vi "binarization.vi"() -> ()   [LabVIEW 2024]
uses:
  <vilib>/vision/NI_Vision_Development_Module.lvlib
panel:
  out "SEGMENTED":T1(plugin-control)
  out "error out 4":errorcluster
  out "RED-PLANE":T1(plugin-control)
  out "EQHP":T1(plugin-control)
  out "EQ-LAP":T1(plugin-control)
  out "LAPLAZ":T2(graph)
  out "HIGHP":T2(graph)
  out "LAPL":T1(plugin-control)
  out "FILL LAPLAZ":T1(plugin-control)
  in  "Range 3":cluster{"Lower value":sgl, "Upper value":sgl}={"Lower value"=128.0, "Upper value"=255.0} {"Upper value" format="%.2f"; "Lower value" format="%.2f"}
  out "HIGHPASS":T1(plugin-control)
  out "FILL HIGHPASS":T1(plugin-control)
  in  "Range 2":cluster{"Lower value":sgl, "Upper value":sgl}={"Lower value"=128.0, "Upper value"=255.0} {"Upper value" format="%.2f"; "Lower value" format="%.2f"}
  out "GAUSS":T1(plugin-control)
  out "High-pass":T1(plugin-control)
  out "Laplacian":T1(plugin-control)
  out "Gray":T1(plugin-control)
  out "Equalized":T1(plugin-control)
  out "Waveform Graph 2":T2(graph)
  out "Waveform Graph":T2(graph)
  out "Threshold":T1(plugin-control)
  out "EQUALI":T1(plugin-control)
  out "FILL EQUA":T1(plugin-control)
  in  "Range":cluster{"Lower value":sgl, "Upper value":sgl}={"Lower value"=128.0, "Upper value"=255.0} {"Upper value" format="%.2f"; "Lower value" format="%.2f"}
  out "error out 2":errorcluster
  in  "stop":bool
  out "Select ROI ->  IZQUIERDO":T1(plugin-control)
  out "Ojo Izquierdo":T1(plugin-control)
  out "error out":errorcluster
  out "error out 3":errorcluster
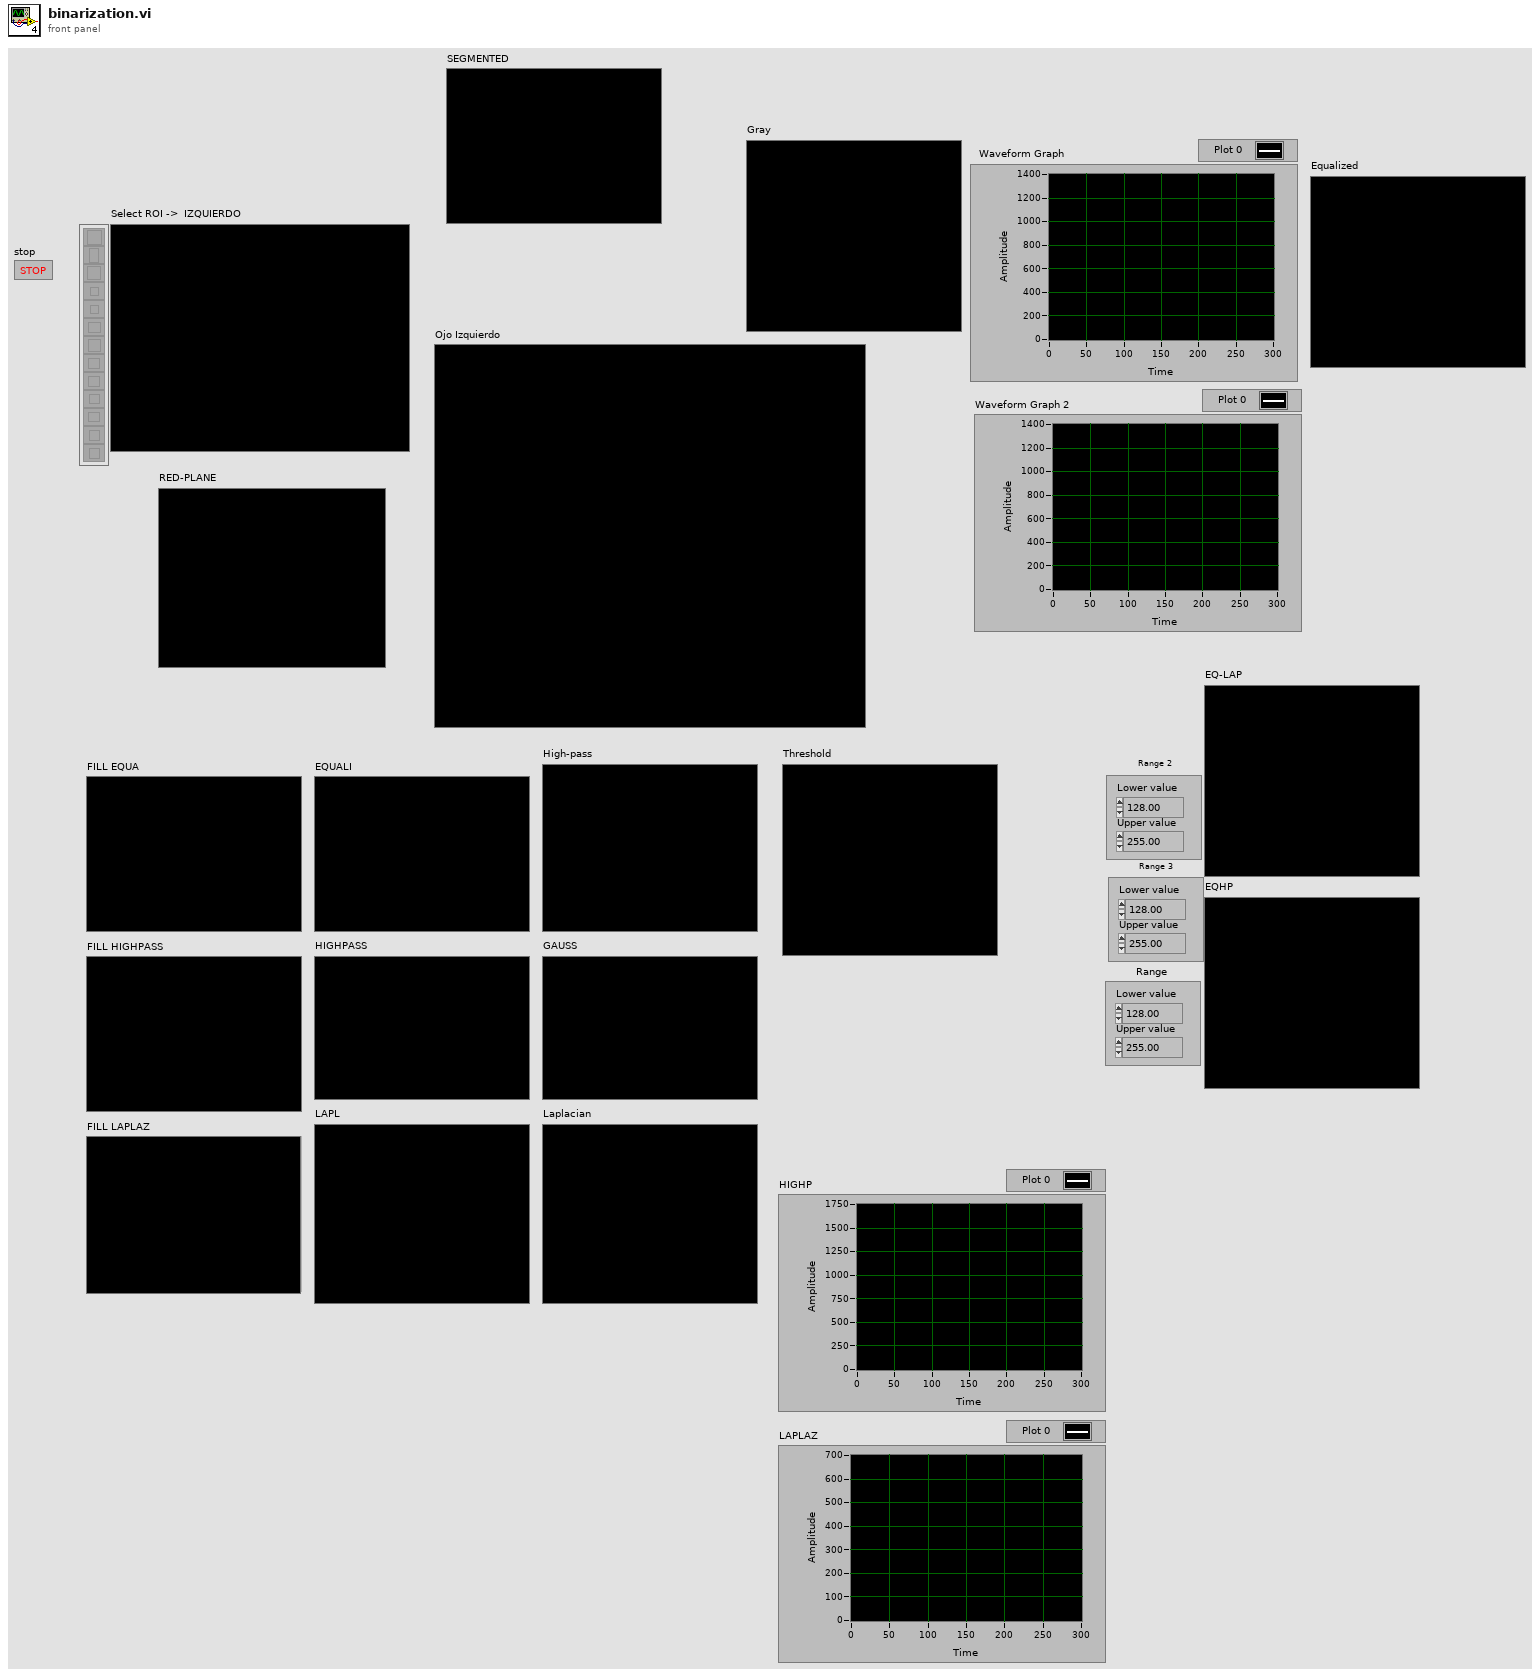
[diagram p1: front panel]
types:
  T1 = typedef "IMAQ Image.ctl" = refnum<image>
  T2 = cluster{"Starting Value":sgl, "Incremental Value":sgl, "Histogram":u32[]}
  T3 = typedef "Image Type" = u32
  T4 = cluster{"Global Rectangle":i32[], "Contours":cluster{"Contour Type":u32, "ROI Type":u32, "Points":i32[]}[]}
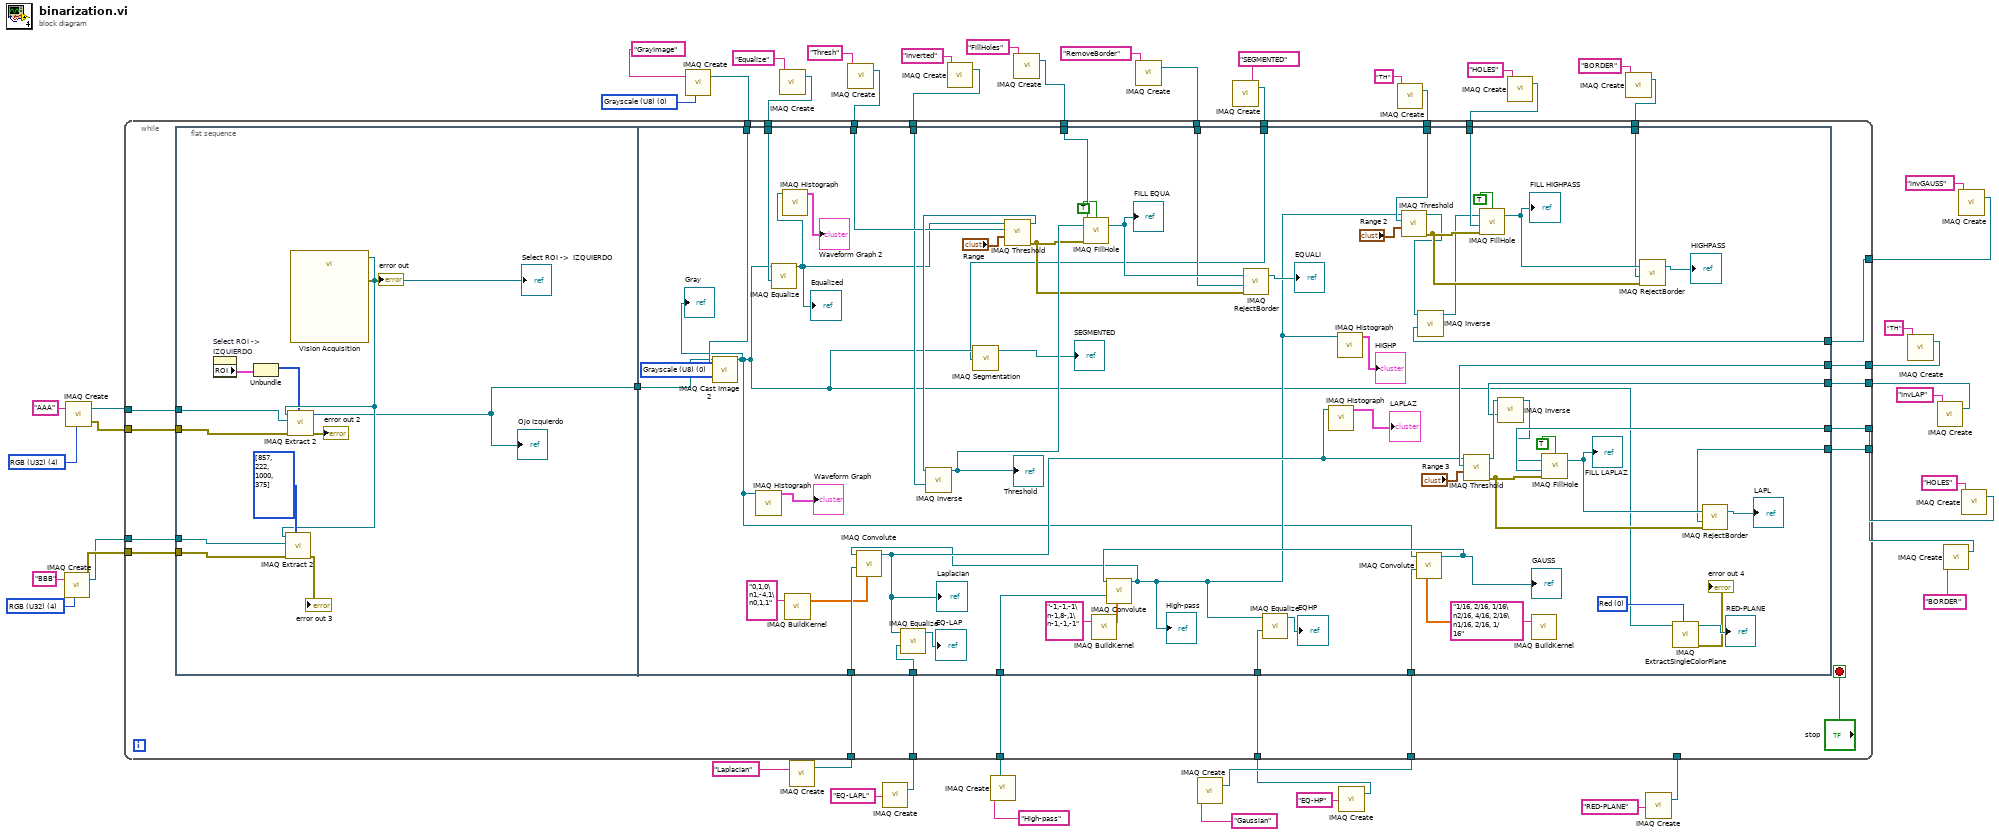
[diagram p0: block diagram]
diagram:
  w42 = T3 0 items=["Grayscale (U8)", "Grayscale (I16)", "Grayscale (SGL)", "Complex (CSG)", "RGB (U32)", "HSL (U32)", "RGB (U64)", "Grayscale (U16)"] ("Image Type")
  w46 = T3 4 items=["Grayscale (U8)", "Grayscale (I16)", "Grayscale (SGL)", "Complex (CSG)", "RGB (U32)", "HSL (U32)", "RGB (U64)", "Grayscale (U16)"] ("Image Type")
  w44 = T3 4 items=["Grayscale (U8)", "Grayscale (I16)", "Grayscale (SGL)", "Complex (CSG)", "RGB (U32)", "HSL (U32)", "RGB (U64)", "Grayscale (U16)"] ("Image Type")
  n1 = call "IMAQ Create"("Image Name"="BBB", "Image Type"=w46) -> ("New Image"=w50:T1, "error out"=w51:errorcluster)  [unwired: 3 in]
  n2 = call "IMAQ Create"("Image Name"="AAA", "Image Type"=w44) -> ("New Image"=w48:T1, "error out"=w49:errorcluster)  [unwired: 3 in]
  n3 = call "IMAQ Create"("Image Name"="GrayImage", "Image Type"=w42) -> ("New Image"=w41:T1)  [unwired: 3 in, 1 out]
  n4 = call "IMAQ Create"("Image Name"="Equalize") -> ("New Image"=w31:T1)  [unwired: 4 in, 1 out]
  n5 = call "IMAQ Create"("Image Name"="Laplacian") -> ("New Image"=w29:T1)  [unwired: 4 in, 1 out]
  n6 = call "IMAQ Create"("Image Name"="Thresh") -> ("New Image"=w36:T1)  [unwired: 4 in, 1 out]
  n7 = call "IMAQ Create"("Image Name"="EQ-LAPL") -> ("New Image"=w7:T1)  [unwired: 4 in, 1 out]
  n8 = call "IMAQ Create"("Image Name"="Inverted") -> ("New Image"=w35:T1)  [unwired: 4 in, 1 out]
  n9 = call "IMAQ Create"("Image Name"="High-pass") -> ("New Image"=w27:T1)  [unwired: 4 in, 1 out]
  n10 = call "IMAQ Create"("Image Name"="FillHoles") -> ("New Image"=w34:T1)  [unwired: 4 in, 1 out]
  n11 = call "IMAQ Create"("Image Name"="RemoveBorder") -> ("New Image"=w33:T1)  [unwired: 4 in, 1 out]
  n12 = call "IMAQ Create"("Image Name"="Gaussian") -> ("New Image"=w25:T1)  [unwired: 4 in, 1 out]
  n13 = call "IMAQ Create"("Image Name"="SEGMENTED") -> ("New Image"=w1:T1)  [unwired: 4 in, 1 out]
  n14 = call "IMAQ Create"("Image Name"="EQ-HP") -> ("New Image"=w5:T1)  [unwired: 4 in, 1 out]
  n15 = call "IMAQ Create"("Image Name"="TH") -> ("New Image"=w21:T1)  [unwired: 4 in, 1 out]
  n16 = call "IMAQ Create"("Image Name"="HOLES") -> ("New Image"=w20:T1)  [unwired: 4 in, 1 out]
  n17 = call "IMAQ Create"("Image Name"="BORDER") -> ("New Image"=w19:T1)  [unwired: 4 in, 1 out]
  n18 = call "IMAQ Create"("Image Name"="RED-PLANE") -> ("New Image"=w3:T1)  [unwired: 4 in, 1 out]
  n19 = call "IMAQ Create"("Image Name"="TH") -> ("New Image"=w15:T1)  [unwired: 4 in, 1 out]
  n20 = call "IMAQ Create"("Image Name"="invLAP") -> ("New Image"=w11:T1)  [unwired: 4 in, 1 out]
  n21 = call "IMAQ Create"("Image Name"="BORDER") -> ("New Image"=w13:T1)  [unwired: 4 in, 1 out]
  n22 = call "IMAQ Create"("Image Name"="invGAUSS") -> ("New Image"=w9:T1)  [unwired: 4 in, 1 out]
  n23 = call "IMAQ Create"("Image Name"="HOLES") -> ("New Image"=w14:T1)  [unwired: 4 in, 1 out]
  n24 = while {
    tunnel: w48 -> [w75]
    tunnel: w49 -> [w76]
    tunnel: w50 -> [w74]
    tunnel: w51 -> [w73]
    tunnel: w41 -> [w72]
    tunnel: w36 -> [w70]
    tunnel: w35 -> [w69]
    tunnel: w34 -> [w68]
    tunnel: w33 -> [w67]
    tunnel: w31 -> [w66]
    tunnel: w29 -> [w65]
    tunnel: w27 -> [w64]
    tunnel: w25 -> [w63]
    tunnel: w21 -> [w62]
    tunnel: w20 -> [w61]
    tunnel: w19 -> [w60]
    tunnel: w15 -> [w59]
    tunnel: w14 -> [w58]
    tunnel: w13 -> [w57]
    tunnel: w11 -> [w56]
    tunnel: w9 -> [w55]
    tunnel: w7 -> [w54]
    tunnel: w5 -> [w53]
    tunnel: w3 -> [_]
    tunnel: w1 -> [w52]
    stop <- "stop" stop-if-true
    n25 = flat-sequence {
      tunnel: w76 -> [w88]
      tunnel: w75 -> [w87]
      tunnel: w74 -> [w85]
      tunnel: w73 -> [w84]
      tunnel: [w80] -> w71
      tunnel: w72 -> [w153]
      tunnel: w71 -> [w152]
      tunnel: w70 -> [w144]
      tunnel: w69 -> [w143]
      tunnel: w68 -> [w142]
      tunnel: w67 -> [w141]
      tunnel: w66 -> [w137]
      tunnel: w65 -> [w135]
      tunnel: w64 -> [w131]
      tunnel: w63 -> [w128]
      tunnel: w62 -> [w121]
      tunnel: w61 -> [w120]
      tunnel: w60 -> [w119]
      tunnel: w59 -> [w112]
      tunnel: w58 -> [w111]
      tunnel: w57 -> [w110]
      tunnel: w56 -> [w105]
      tunnel: w55 -> [w104]
      tunnel: w54 -> [w100]
      tunnel: w53 -> [w96]
      tunnel: w52 -> [w90]
      frame #0 {
        n26 = property on="Select ROI ->  IZQUIERDO" class="ImageControl"() -> ("ROI"=w79:T4)  [unwired: 2 in, 2 out]
        n27 = Unbundle(w79) -> ("Global Rectangle"=w78:i32[])  [unwired: 1 out]
        n28 = call "Vision Acquisition"() -> ("Image Out"=w82:T1, "error out"=→"error out":errorcluster)  [unwired: 25 in, 1 out]
        "Select ROI ->  IZQUIERDO" <- w82
        n29 = call "IMAQ Extract 2"("Optional Rectangle"=i32[] [857, 222, 1000, 375], "error in (no error)"=w84, "Image Dst"=w85, "Image Src"=w82) -> ("error out"=→"error out 3":errorcluster)  [unwired: 6 in, 1 out]
        n30 = call "IMAQ Extract 2"("Optional Rectangle"=w78, "error in (no error)"=w88, "Image Dst"=w87, "Image Src"=w82) -> ("error out"=→"error out 2":errorcluster, "Image Dst Out"=w80:T1)  [unwired: 6 in]
        "Ojo Izquierdo" <- w80
      }
      frame #1 {
        w95 = 0 items=["Red", "Green", "Blue", "Hue", "Saturation", "Luminance", "Value", "Intensity"] ("Color Plane")
        w151 = T3 0 items=["Grayscale (U8)", "Grayscale (I16)", "Grayscale (SGL)", "Complex (CSG)", "RGB (U32)", "HSL (U32)", "RGB (U64)", "Grayscale (U16)"] ("Image Type")
        n31 = call "IMAQ Cast Image 2"("Image Src"=w152, "Image Dst"=w153, "Image Type"=w151) -> ("Image Dst Out"=w92:T1)  [unwired: 11 in, 1 out]
        "Gray" <- w92
        n32 = call "IMAQ Histograph"("Image"=w92) -> ("Histogram Graph"=→"Waveform Graph":T2)  [unwired: 7 in, 3 out]
        n33 = call "IMAQ Equalize"("Image Dst"=w137, "Image Src"=w92) -> ("Image Dst Out"=w118:T1)  [unwired: 8 in, 1 out]
        "Equalized" <- w118
        n34 = call "IMAQ Histograph"("Image"=w118) -> ("Histogram Graph"=→"Waveform Graph 2":T2)  [unwired: 7 in, 3 out]
        n35 = call "IMAQ BuildKernel"("Kernel String"="0,1,0\n1,-4,1\n0,1,1") -> ("Kernel"=w134:sgl[][])  [unwired: 4 in, 1 out]
        n36 = call "IMAQ Segmentation"("Image Dst"=w90, "Image Src"=w92) -> ("Image Dst Out"=→"SEGMENTED":T1)  [unwired: 2 in, 1 out]
        n37 = call "IMAQ Threshold"("Range"="Range", "Image Dst"=w144, "Image Src"=w118) -> ("error out"=w148:errorcluster, "Image Dst Out"=w149:T1)  [unwired: 7 in]
        n38 = call "IMAQ Inverse"("Image Dst"=w143, "Image Src"=w149) -> ("Image Dst Out"=w150:T1)  [unwired: 8 in, 1 out]
        "Threshold" <- w150
        n39 = call "IMAQ FillHole"("error in (no error)"=w148, "Image Dst"=w142, "Image Src"=w150, "Connectivity 4/8 (8)"=TRUE) -> ("Image Dst Out"=w147:T1)  [unwired: 2 in, 1 out]
        "FILL EQUA" <- w147
        n40 = call "IMAQ BuildKernel"("Kernel String"="-1,-1,-1\n-1,8-,1\n-1,-1,-1") -> ("Kernel"=w132:sgl[][])  [unwired: 4 in, 1 out]
        n41 = call "IMAQ RejectBorder"("error in (no error)"=w148, "Image Dst"=w141, "Image Src"=w147) -> ("Image Dst Out"=→"EQUALI":T1)  [unwired: 3 in, 1 out]
        n42 = call "IMAQ BuildKernel"("Kernel String"="1/16, 2/16, 1/16\n2/16, 4/16, 2/16\n1/16, 2/16, 1/16") -> ("Kernel"=w129:sgl[][])  [unwired: 4 in, 1 out]
        n43 = call "IMAQ Convolute"("Kernel"=w129, "Image Dst"=w128, "Image Src"=w92) -> ("Image Dst Out"=w127:T1)  [unwired: 7 in, 1 out]
        "GAUSS" <- w127
        n44 = call "IMAQ Convolute"("Kernel"=w132, "Image Dst"=w131, "Image Src"=w127) -> ("Image Dst Out"=w97:T1)  [unwired: 7 in, 1 out]
        "High-pass" <- w97
        n45 = call "IMAQ Convolute"("Kernel"=w134, "Image Dst"=w135, "Image Src"=w97) -> ("Image Dst Out"=w101:T1)  [unwired: 7 in, 1 out]
        "Laplacian" <- w101
        n46 = call "IMAQ Equalize"("Image Dst"=w100, "Image Src"=w101) -> ("Image Dst Out"=→"EQ-LAP":T1)  [unwired: 8 in, 1 out]
        n47 = call "IMAQ Equalize"("Image Dst"=w96, "Image Src"=w97) -> ("Image Dst Out"=→"EQHP":T1)  [unwired: 8 in, 1 out]
        n48 = call "IMAQ Histograph"("Image"=w101) -> ("Histogram Graph"=→"LAPLAZ":T2)  [unwired: 7 in, 3 out]
        n49 = call "IMAQ Histograph"("Image"=w97) -> ("Histogram Graph"=→"HIGHP":T2)  [unwired: 7 in, 3 out]
        n50 = call "IMAQ Threshold"("Range"="Range 2", "Image Dst"=w121, "Image Src"=w97) -> ("error out"=w126:errorcluster, "Image Dst Out"=w108:T1)  [unwired: 7 in]
        n51 = call "IMAQ Inverse"("Image Dst"=w104, "Image Src"=w108) -> ("Image Dst Out"=w109:T1)  [unwired: 8 in, 1 out]
        n52 = call "IMAQ Threshold"("Range"="Range 3", "Image Dst"=w112, "Image Src"=w101) -> ("error out"=w117:errorcluster, "Image Dst Out"=w106:T1)  [unwired: 7 in]
        n53 = call "IMAQ FillHole"("error in (no error)"=w126, "Image Dst"=w120, "Image Src"=w109, "Connectivity 4/8 (8)"=TRUE) -> ("Image Dst Out"=w125:T1)  [unwired: 2 in, 1 out]
        "FILL HIGHPASS" <- w125
        n54 = call "IMAQ Inverse"("Image Dst"=w105, "Image Src"=w106) -> ("Image Dst Out"=w107:T1)  [unwired: 8 in, 1 out]
        n55 = call "IMAQ FillHole"("error in (no error)"=w117, "Image Dst"=w111, "Image Src"=w107, "Connectivity 4/8 (8)"=TRUE) -> ("Image Dst Out"=w116:T1)  [unwired: 2 in, 1 out]
        "FILL LAPLAZ" <- w116
        n56 = call "IMAQ RejectBorder"("error in (no error)"=w126, "Image Dst"=w119, "Image Src"=w125) -> ("Image Dst Out"=→"HIGHPASS":T1)  [unwired: 3 in, 1 out]
        n57 = call "IMAQ ExtractSingleColorPlane"("Color Plane"=w95, "Image Src"=w92) -> ("error out"=→"error out 4":errorcluster, "Image Dst Out"=→"RED-PLANE":T1)  [unwired: 8 in]
        n58 = call "IMAQ RejectBorder"("error in (no error)"=w117, "Image Dst"=w110, "Image Src"=w116) -> ("Image Dst Out"=→"LAPL":T1)  [unwired: 3 in, 1 out]
      }
    }
  }
